vi "FTW-Example-SlasdClient-Core-Initialize.vi"(0 "Initialization Sequence":string, 5 "FTW Actor Instance Configuration":string, 11 "error in (no error)":errorcluster) -> (4 "Actor Template-Core out":refnum<class "FTW-Example-SlasdClient-Core.lvclass">, 6 "Incoming Requests":refnum<event-registration>, 8 "SLASD Subscription":refnum<event-registration>, 15 "error out":errorcluster)   [LabVIEW 2018, in "FTW-Example-SlasdClient-Core.lvclass"]
uses:
  FTW-Example-SlasdClient-Core.lvclass
  source/CodeGen/JSON Deserialize/FTW-JSON-Deserialize.xnode
  SLASD/FTW-Example-SLASD.lvclass
  source/CodeGen/JSON Deserialize/FTW-JSON-Core-GetFlattenedValue.vi
  source/Reflection/FTW-Reflection-Type.vi
  source/JSON/core/FTW-JSON-Core-EncodingFlags.vi
  source/JSON/FTW-JSON-Parse.vi
  source/actor/Message/Request/FTW-Message-IncomingRequest.lvclass
  C:/Jobs/Featherweight/featherweight-2018/source/actor/Message/Base/FTW-Message.lvclass
  source/actor/Message/Base/FTW-Message.lvclass
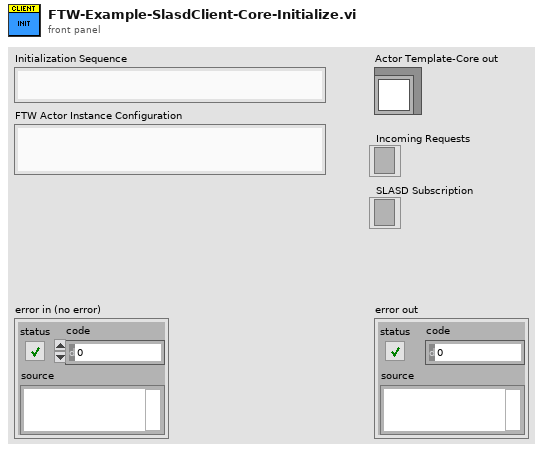
[diagram p1: front panel]
types:
  T1 = cluster{"Incoming Requests":refnum<event-registration>, "Local Messages":refnum<event-registration>, "Subscriber Registration":refnum<event-registration>}
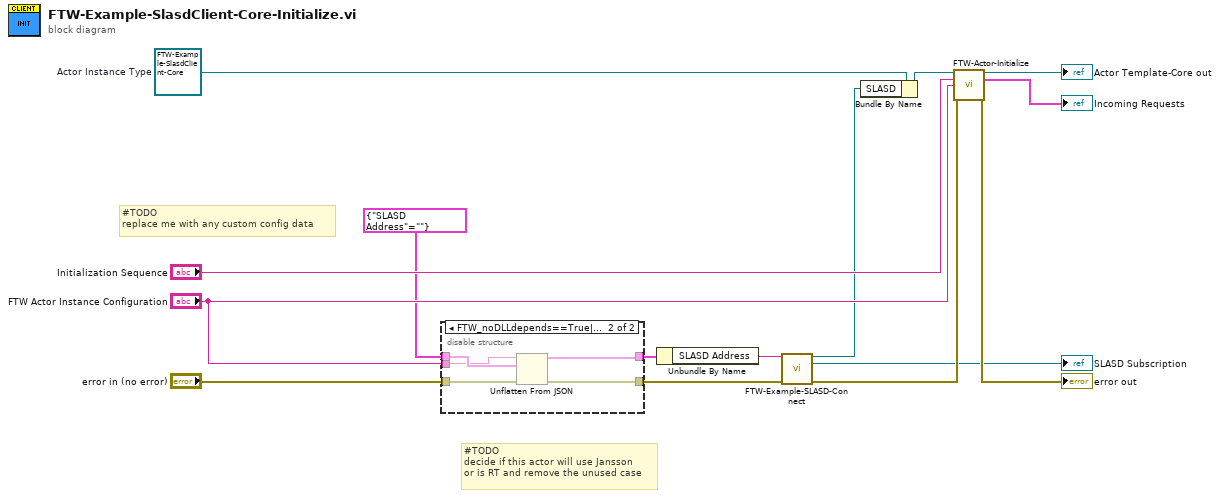
[diagram p0: block diagram]
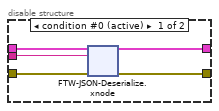
[diagram p2: hidden frame]
diagram:
  w6 = refnum<class "FTW-Example-SlasdClient-Core.lvclass"> refnum  # Actor Instance Type
  # "#TODO\ndecide if this actor will use Jansson\nor is RT and remove the unused case"
  # "#TODO\nreplace me with any custom config data"
  n1 = disable-structure shown="FTW_noDLLdepends==True||TARGET_TYPE==RT" {
    disable-tunnel: "error in (no error)" -> [w20 w37]
    disable-tunnel: [w19 w36] -> w10
    disable-tunnel: "FTW Actor Instance Configuration" -> [w18 w34]
    disable-tunnel: cluster{"SLASD Address":string} {"SLASD Address"=""} ("Type and Defaults") -> [w17 w35]
    disable-tunnel: [w16 w33] -> w7
    frame condition #0 (active) {
      n2 = xnode "FTW-JSON-Deserialize.xnode"("Type and Defaults"=w17, "JSON String"=w18, "error in"=w20) -> ("Values"=w16:cluster{"SLASD Address":string}, "error out"=w19:errorcluster)
    }
    frame condition #1 {
      n3 = Unflatten From JSON(JSON string=w34, type and defaults=w35, error in (no error)=w37) -> (value=w33:cluster{"SLASD Address":string}, error out=w36:errorcluster)  [unwired: 4 in]
    }
  }
  n4 = Unbundle By Name(w7) -> ("SLASD Address"=w4:string)
  n5 = call "FTW-Example-SLASD-Connect.vi"("IP Address"=w4, "error in"=w10) -> ("FTW Actor Connector"=w2:refnum<class "FTW-Example-SLASD.lvclass">, "Subscription Registration Refnum"=→"SLASD Subscription":refnum<event-registration>, "error out"=w5:errorcluster)  [unwired: 11 in]
  n6 = Bundle By Name(cluster=w6, "SLASD"=w2) -> (w3:refnum<class "FTW-Example-SlasdClient-Core.lvclass">)
  n7 = call-dynamic "FTW-Actor-Initialize.vi"("FTW Actor Instance Type"=w3, "Initialization Job Sequence"="Initialization Sequence", "Actor Instance Configuration"="FTW Actor Instance Configuration", "error in"=w5) -> ("FTW Actor Instance"=→"Actor Template-Core out":refnum<class "FTW-Example-SlasdClient-Core.lvclass">, "Event Refnums"=→"Incoming Requests":T1, "error out"=→"error out":errorcluster)  [unwired: 9 in]
